vi "Test a single relay.vi"() -> ()   [LabVIEW 2018, in "MB Relay.lvlib"]
uses:
  MB Relay.lvlib
  <vilib>/NI/Modbus Library/API/Modbus API.lvclass/Modbus API.ctl
  <vilib>/NI/Modbus Library/Transmission Data Unit/Transmission Data Unit.lvclass/Transmission Data Unit.ctl
  <vilib>/NI/Modbus Library/Transmission Data Unit/Write Unit ID.vi
  <vilib>/NI/Modbus Library/API/Read Transmission Data Unit.vi
  <vilib>/NI/Modbus Library/API/Write Transmission Data Unit.vi
  <vilib>/NI/Modbus Library/API/Master/Modbus Master.lvclass
  C:/Program Files (x86)/National Instruments/LabVIEW 2018/vi.lib/NI/Modbus Library/API/Modbus API.lvclass
  <vilib>/NI/Modbus Library/API/Wrapper/Create Serial Master.vi
  <vilib>/NI/Modbus Library/API/Wrapper/API Main.lvlib
panel:
  out "counter":u16
  in  "Relay Positions":u16 format="%b"
  in  "Stop Button":bool
  in  "VISA resource name":refnum<visa-resource-name>
  in  "error in":errorcluster
  out "error out":errorcluster
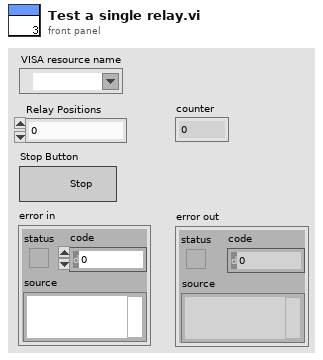
[diagram p1: front panel]
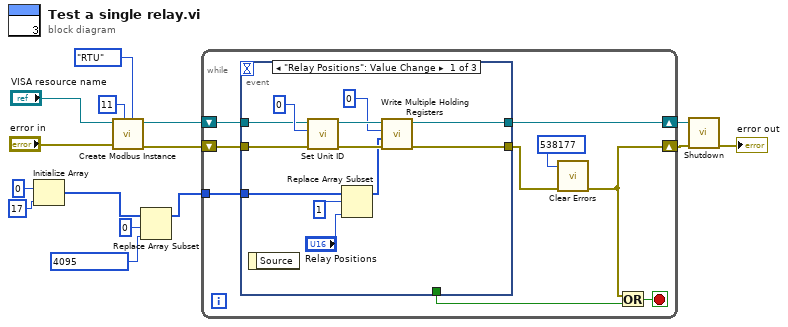
[diagram p0: block diagram]
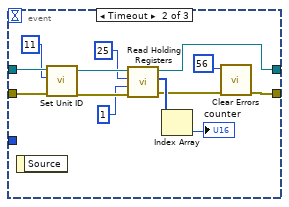
[diagram p2: hidden frame]
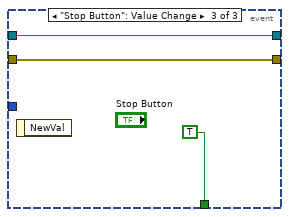
[diagram p3: hidden frame]
diagram:
  n1 = Initialize Array(u16 0 ("element"), 17 ("dimension size")) -> (w2:u16[])
  n2 = call-poly <vilib>:"Create Modbus Instance.vi"("serial type"=enum16{"RTU", "ASCII"}."RTU", "unit ID"=u8 11, "error in"="error in", "VISA resource name"="VISA resource name") -> ("error out"=w15:errorcluster, "serial master instance"=w13:refnum<class "Modbus Master.lvclass">)  [unwired: 6 in]
  n3 = Replace Array Subset(array=w2, new element=u16 4095 ("new element/subarray"), index=0) -> (w1:u16[])
  n4 = while {
    shift-right: [w17] -> w11
    shift-left: w15 -> [w24]
    shift-right: [w22] -> w9
    shift-left: w13 -> [w23]
    tunnel: w1 -> [w16]
    stop <- w20 stop-if-true
    n5 = event shown="[0] \"Relay Positions\": Value Change" {
      selector: _ -> [_ _ _]
      dyn-events: _ -> [_ _ _]
      timeout: _ -> [_ _ _]
      tunnel: w24 -> [w32 w47 w50]
      tunnel: w23 -> [w31 w49 w51]
      tunnel: [w30 w37 w50] -> w18
      tunnel: [_ _ TRUE] -> w21
      tunnel: [w29 w38 w51] -> w22
      tunnel: w16 -> [w28 _ _]
      event "Relay Positions": Value Change {
        n6 = event-data() -> ()  [unwired: 1 in, 1 out]
        n7 = call <vilib>:"Set Unit ID.vi"("error in"=w32, "unit ID"=u8 0, "Modbus master in"=w31) -> ("error out"=w33:errorcluster, "Modbus master out"=w36:refnum<class "Modbus Master.lvclass">)  [unwired: 7 in]
        n8 = Replace Array Subset(array=w28, new element="Relay Positions", index=1) -> (w25:u16[])
        n9 = call-dynamic "Write Multiple Holding Registers.vi"("error in"=w33, "registers to write"=w25, "starting address"=u16 0 ("address"), "Modbus master in"=w36) -> ("error out"=w30:errorcluster, "Modbus master out"=w29:refnum<class "Modbus Master.lvclass">)  [unwired: 6 in]
      }
      event Timeout {
        n10 = event-data() -> ()  [unwired: 1 in, 1 out]
        n11 = call <vilib>:"Set Unit ID.vi"("error in"=w47, "unit ID"=u8 11, "Modbus master in"=w49) -> ("error out"=w45:errorcluster, "Modbus master out"=w46:refnum<class "Modbus Master.lvclass">)  [unwired: 7 in]
        n12 = call-dynamic "Read Holding Registers.vi"("error in"=w45, "number of inputs"=u16 1, "starting address"=u16 25, "Modbus master in"=w46) -> ("error out"=w39:errorcluster, "register values"=w42:u16[], "Modbus master out"=w38:refnum<class "Modbus Master.lvclass">)  [unwired: 5 in]
        n13 = Index Array(array=w42) -> (element=→"counter":u16)  [unwired: 1 in]
        n14 = call <vilib>:"Clear Errors.vi"("error in (no error)"=w39, "specific error code to clear (0: all)"=56) -> ("error out"=w37:errorcluster)  [unwired: 4 in, 1 out]
      }
      event "Stop Button": Value Change {
        n15 = event-data() -> ()  [unwired: 1 in, 1 out]
      }
    }
    n16 = call <vilib>:"Clear Errors.vi"("error in (no error)"=w18, "specific error code to clear (0: all)"=538177) -> ("error out"=w17:errorcluster)  [unwired: 4 in, 1 out]
    n17 = Or(x=w17, y=w21) -> (x .or. y?=w20:bool)
  }
  n18 = call-dynamic "Shutdown.vi"("error in"=w11, "Modbus master in"=w9) -> ("error out"=→"error out":errorcluster)  [unwired: 9 in]
